vi "Actor Core.vi"(8 "error in":errorcluster, 11 "HSplittedX4 in":refnum<class "HSplittedX4.lvclass">) -> (0 "error out":errorcluster, 3 "Actor out":refnum<class "Actor.lvclass">)   [LabVIEW 2020, in "HSplittedX4.lvlib" / "HSplittedX4.lvclass"]
doc: "The user interface for this panel.\n\n----\nPlease see the following web address for additional documentation and tutorial information:\nhttp://www.mooregoodideas.com/mgi-panel-manager/\n\nAuthor: Derek Trepanier\n\nCopyright (c) 2018, Moore Good Ideas, Inc.\n\nAll rights reserved.\n\nRedistribution and use in source and binary forms, with or without modification, are permitted provided that the following conditions are met:\n\n * Redistributions of source code must retain the above copyright notice, this list of conditions and the following disclaimer.\n * Redistributions in binary form must reproduce the above copyright notice, this list of conditions and the following disclaimer in the documentation and/or other materials provided with the distribution.\n * Neither the name of Moore Good Ideas, Inc. nor the names of its contributors may be used to endorse or promote products derived from this software without specific prior written permission.\n\nTHIS SOFTWARE IS PROVIDED BY THE COPYRIGHT HOLDERS AND CONTRIBUTORS \"AS IS\" AND ANY EXPRESS OR IMPLIED WARRANTIES, INCLUDING, BUT NOT LIMITED TO, THE IMPLIED WARRANTIES OF MERCHANTABILITY AND FITNESS FOR A PARTICULAR PURPOSE ARE DISCLAIMED. IN NO EVENT SHALL THE COPYRIGHT OWNER OR CONTRIBUTORS BE LIABLE FOR ANY DIRECT, INDIRECT, INCIDENTAL, SPECIAL, EXEMPLARY, OR CONSEQUENTIAL DAMAGES (INCLUDING, BUT NOT LIMITED TO, PROCUREMENT OF SUBSTITUTE GOODS OR SERVICES; LOSS OF USE, DATA, OR PROFITS; OR BUSINESS INTERRUPTION) HOWEVER CAUSED AND ON ANY THEORY OF LIABILITY, WHETHER IN CONTRACT, STRICT LIABILITY, OR TORT (INCLUDING NEGLIGENCE OR OTHERWISE) ARISING IN ANY WAY OUT OF THE USE OF THIS SOFTWARE, EVEN IF ADVISED OF THE POSSIBILITY OF SUCH DAMAGE."
uses:
  HSplittedX4.lvclass
  <vilib>/ActorFramework/Actor/Actor.lvclass
  HSplitted/HSplitted/HSplitted.lvclass
  HSplittedX4.lvclass/HSplittedX4.ctl
  <vilib>/MGI/Panel Manager/Panel Actor/Panel Actor/Panel Actor.lvclass
  <vilib>/ActorFramework/Stop Msg/Stop Msg.lvclass
  C:/Users/Test/Git/MGIPanelActors-Exploration/src/HSplitted/HSplitted/HSplitted.lvclass
  C:/Program Files (x86)/National Instruments/LabVIEW 2020/vi.lib/MGI/Panel Manager/Panel Actor/Panel Actor/Panel Actor.lvclass
  C:/Program Files (x86)/National Instruments/LabVIEW 2020/vi.lib/MGI/Monitored Actor/Monitored Actor/Monitored Actor/Monitored Actor.lvclass
  C:/Program Files (x86)/National Instruments/LabVIEW 2020/vi.lib/ActorFramework/Actor/Actor.lvclass
  C:/Users/Test/Git/MGIPanelActors-Exploration/src/HSplittedX4/HSplittedX4/HSplittedX4.lvclass
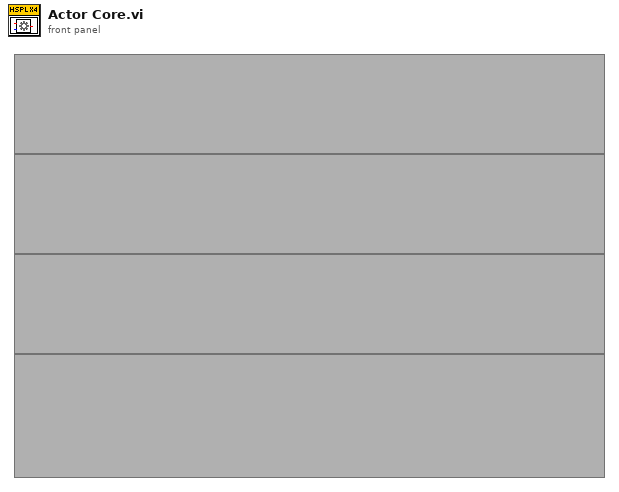
[diagram p1: front panel]
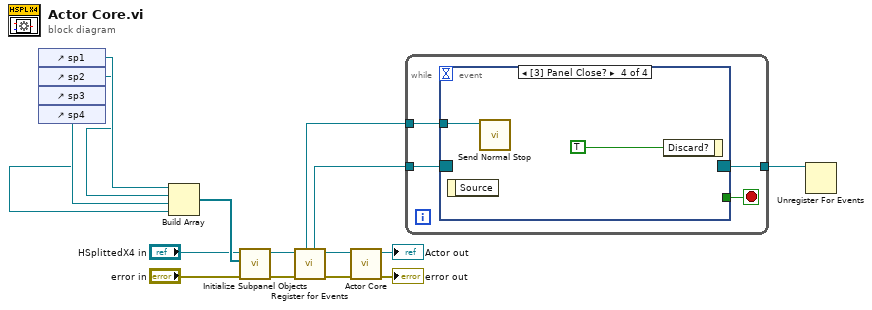
[diagram p0: block diagram]
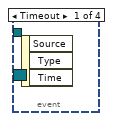
[diagram p2: hidden frame]
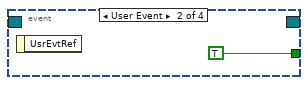
[diagram p3: hidden frame]
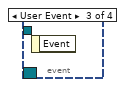
[diagram p4: hidden frame]
diagram:
  n1 = control-ref of="sp1"() -> (w4:refnum<vi>)
  n2 = control-ref of="sp2"() -> (w3:refnum<vi>)
  n3 = control-ref of="sp3"() -> (w2:refnum<vi>)
  n4 = control-ref of="sp4"() -> (w1:refnum<vi>)
  n5 = Build Array(w4, w3, w2, w1) -> (w12:refnum<vi>[])
  n6 = call "Initialize Subpanel Objects.vi"("error in (no error)"="error in", "SubPanelRefs"=w12, "HSplitted in"="HSplittedX4 in") -> ("error out"=w10:errorcluster, "HSplitted out"=w8:refnum<class "HSplittedX4.lvclass">)  [unwired: 7 in]
  n7 = call <vilib>:"Register for Events.vi"("Error In"=w10, "Panel Actor in"=w8) -> ("Error Out"=w6:errorcluster, "Panel Actor out"=w7:refnum<class "HSplittedX4.lvclass">, "Pnl Actor"=w13:refnum<event-registration>, "Self Enqueuer"=w11:refnum<class "Message Enqueuer.lvclass">)  [unwired: 6 in]
  n8 = call-parent "Actor Core.vi"("error in"=w6, "Panel Actor in"=w7) -> ("error out"=→"error out":errorcluster, "Actor out"=→"Actor out":refnum<class "Actor.lvclass">)  [unwired: 8 in]
  n9 = while {
    tunnel: w13 -> [w20]
    tunnel: w11 -> [w19]
    tunnel: [w17] -> w14
    stop <- w18 stop-if-true
    n10 = event shown="[3] Panel Close?" {
      selector: w20 -> [_ _ _ _]
      dyn-events: [_ _ _ _] -> w17
      timeout: _ -> [_ _ _ _]
      tunnel: w19 -> [_ _ _ w23]
      tunnel: [_ TRUE _ _] -> w18
      event Timeout {
        n11 = event-data() -> ()  [unwired: 1 in, 3 out]
      }
      event User Event {
        n12 = event-data() -> ()  [unwired: 1 in, 1 out]
      }
      event User Event {
        n13 = event-data() -> ()  [unwired: 1 in, 1 out]
      }
      event Panel Close? {
        n14 = event-data() -> ()  [unwired: 1 in, 1 out]
        n15 = call <vilib>:"Send Normal Stop.vi"("Message Enqueuer"=w23) -> ()  [unwired: 10 in, 1 out]
        n16 = event-data("Discard?"=TRUE) -> ()  [unwired: 1 in, 1 out]
      }
    }
  }
  n17 = Unregister For Events(event registration refnum=w14) -> ()  [unwired: 1 in, 1 out]
